vi "Crash_check (SubVI).vi"(8 "error in (no error)":errorcluster, 11 "Application in":refnum<vi>) -> (0 "error out":errorcluster, 1 "crashed?":bool, 3 "Application out":refnum<vi>)   [LabVIEW 2014]
uses:
  <userlib>/Nanonis Prog Interface V5/Nanonis Prog Interface.lvlib
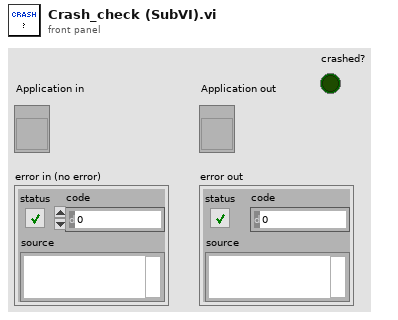
[diagram p1: front panel]
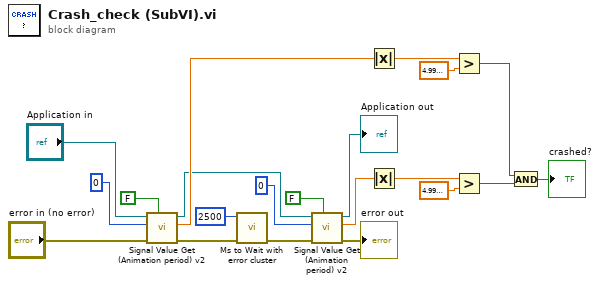
[diagram p0: block diagram]
diagram:
  n1 = call <userlib>:"Signal Value Get (Animation period) v2.vi"("Wait for newest data (F=False)"=FALSE, "error in (no error)"="error in (no error)", "Signal index (0-79)"=i8 0, "Application ref in"="Application in") -> ("error out"=w13:errorcluster, "Signal value"=w16:sgl, "Application ref out"=w5:refnum<vi>)  [unwired: 4 in]
  n2 = call <userlib>:"Ms to Wait with error cluster.vi"("error in (no error)"=w13, "milliseconds to wait"=u32 2500) -> ("error out"=w7:errorcluster)  [unwired: 4 in, 1 out]
  n3 = call <userlib>:"Signal Value Get (Animation period) v2.vi"("Wait for newest data (F=False)"=FALSE, "error in (no error)"=w7, "Signal index (0-79)"=i8 0, "Application ref in"=w5) -> ("error out"=→"error out":errorcluster, "Signal value"=w9:sgl, "Application ref out"=→"Application out":refnum<vi>)  [unwired: 4 in]
  n4 = Absolute Value(x=w16) -> (abs(x)=w17:sgl)
  n5 = Absolute Value(x=w9) -> (abs(x)=w10:sgl)
  n6 = Greater?(x=w17, y=sgl 5e-09) -> (0:w14:bool)
  n7 = Greater?(x=w10, y=sgl 5e-09) -> (0:w2:bool)
  n8 = And(x=w14, y=w2) -> (x .and. y?=→"crashed?":bool)
